vi "Stop Tracking.vi"(8 "error in (no error)":errorcluster, 10 "Tracker Type":refnum<class "Data Tracker Msg.lvclass">, 11 "Data Tracker in":refnum<class "Data Tracker.lvclass">) -> (0 "error out":errorcluster, 1 "Start Time":timestamp, 2 "Data":refnum<class "Data.lvclass">[](array[class]), 3 "Data Tracker out":refnum<class "Data Tracker.lvclass">, 5 "Duration(s)":dbl)   [LabVIEW 2020, in "Data Tracker.lvlib" / "Data Tracker.lvclass"]
doc: "Clean up the data assosicated with 'Tracker Type', stop tracking the data and cancel subscriptions on the Publisher actor if needed.\nReturn the tracked Data, the Start Time and the tracking Duration."
uses:
  Data Tracker.lvclass
  Messages for this Actor/Data Tracker Msg/Data Tracker Msg.lvclass
  PPL/HDH.Data.Generic.lvlibp/Data.lvclass
  PPL/HDH.Actor Framework.Core.Actor.lvlibp/1abvi3w/vi.lib/ActorFramework/Message Enqueuer/Message Priority.ctl
  Data Tracker.lvclass/Data Tracker.ctl
  PPL/HDH.Actor Framework.Core.Publisher.lvlibp/Publisher Messages/Unsubscribe Msg/Unsubscribe Msg.lvclass
  PPL/HDH.Actor Framework.Core.Actor.lvlibp/1abvi3w/vi.lib/ActorFramework/Message Enqueuer/Message Enqueuer.lvclass
  C:/Current projects/WS/PPL/HDH.Actor Framework.Core.Actor.lvlibp/1abvi3w/vi.lib/ActorFramework/Actor/Actor.lvclass
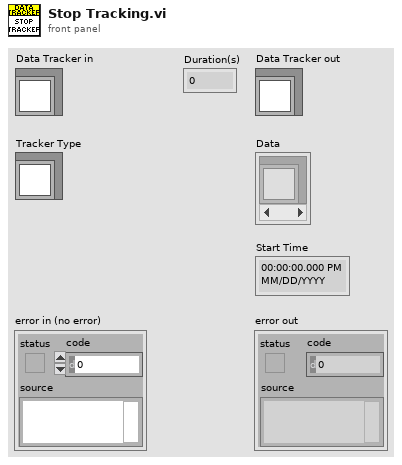
[diagram p1: front panel]
types:
  T1 = typedef "HDH.Actor Framework.Core.Actor.lvlibp/Message Enqueuer.lvclass/Message Priority.ctl" = enum16{"Low", "Normal", "High"}
  T2 = typedef "Data Tracker.lvlib/Data Tracker.lvclass/Ctl_Tracker Element.ctl" = cluster{"Tracker Type":refnum<class "Data Tracker Msg.lvclass">, "Subscriptions":refnum<class "Data.lvclass">[], "Data":refnum<class "Data.lvclass">[], "Size":u32, "Start Time":timestamp}
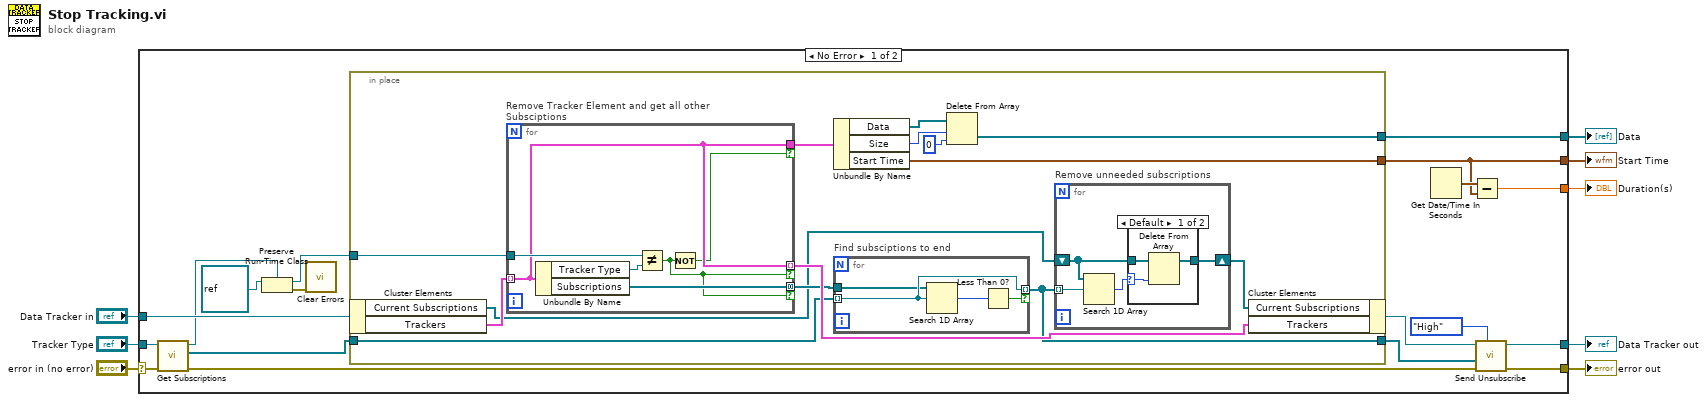
[diagram p0: block diagram]
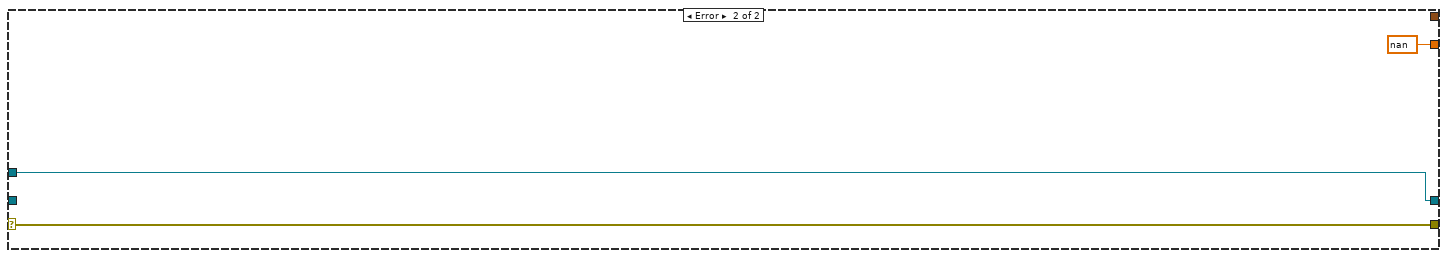
[diagram p3: hidden frame]
diagram:
  n1 = case shown="No Error" "error in (no error)" {
    selector: "error in (no error)" -> [w26 w61]
    tunnel: [w15 w61] -> w7
    tunnel: [w18 w60] -> w5
    tunnel: "Data Tracker in" -> [w24 w60]
    tunnel: "Tracker Type" -> [w22 _]
    tunnel: [w12 _] -> w3
    tunnel: [w10 _] -> w2
    tunnel: [w9 nan] -> w1
    frame No Error {
      n2 = call-dynamic "Get Subscriptions.vi"("error in (no error)"=w26, "Data Tracker Msg in"=w22) -> ("error out"=w16:errorcluster, "Subscriptions"=w20:refnum<class "Data.lvclass">[], "Data Tracker Msg out"=w21:refnum<class "Data Tracker Msg.lvclass">)  [unwired: 7 in]
      n3 = Preserve Run-Time Class(object in=refnum<class> refnum ("LabVIEW Object"), 2:w21) -> (object out=w23:refnum<class "Data Tracker Msg.lvclass">, error out=w25:errorcluster)  [unwired: 1 in]
      n4 = call <vilib>:"Clear Errors.vi"("error in (no error)"=w25) -> ()  [unwired: 5 in, 2 out]
      n5 = in-place {
        in-place-border: w23 -> [w39]
        in-place-border: w20 -> [w37]
        in-place-border: [w33] -> w14
        in-place-border: [w28] -> w12
        in-place-border: [w27] -> w10
        n6 = in-place-cluster #1(w24) -> ("Current Subscriptions"=w35:refnum<class "Data.lvclass">[], "Trackers"=w40:T2[])
        n7 = for "Remove Tracker Element and get all other Subsciptions" {
          tunnel: w40 -> [w55] mode=indexing
          tunnel: w39 -> [w58]
          tunnel: [w55] -> w38 mode=indexing if=w53
          tunnel: [w56] -> w36 mode=concatenating if=w53
          tunnel: [w55] -> w32 if=w54
          n8 = Unbundle By Name(w55) -> ("Tracker Type"=w57:refnum<class "Data Tracker Msg.lvclass">, "Subscriptions"=w56:refnum<class "Data.lvclass">[])
          n9 = Not Equal?(x=w58, y=w57) -> (x != y?=w53:bool)
          n10 = Not(x=w53) -> (.not. x?=w54:bool)
        }
        n11 = Unbundle By Name(w32) -> ("Data"=w31:refnum<class "Data.lvclass">[], "Size"=w29:u32, "Start Time"=w27:timestamp)
        n12 = for "Find subsciptions to end" {
          tunnel: w37 -> [w52] mode=indexing
          tunnel: [w52] -> w33 mode=indexing if=w51
          tunnel: w36 -> [w49]
          n13 = Search 1D Array(1D array=w49, element=w52) -> (index of element=w50:i32)  [unwired: 1 in]
          n14 = Less Than 0?(x=w50) -> (x < 0?=w51:bool)
        }
        n15 = Delete From Array(array=w31, length=w29, index=0) -> (deleted portion=w28:refnum<class "Data.lvclass">[])  [unwired: 1 out]
        n16 = for "Remove unneeded subscriptions" {
          shift-right: [w42] -> w34
          shift-left: w35 -> [w41]
          tunnel: w33 -> [w44] mode=indexing
          n17 = Search 1D Array(1D array=w41, element=w44) -> (index of element=w43:i32)  [unwired: 1 in]
          n18 = case shown="Default" w43 {
            selector: w43 -> [w46 _]
            tunnel: [w45 w48] -> w42
            tunnel: w41 -> [w47 w48]
            frame Default {
              n19 = Delete From Array(array=w47, index=w46) -> (array with subset deleted=w45:refnum<class "Data.lvclass">[])  [unwired: 1 in, 1 out]
            }
            frame -1 {
            }
          }
        }
        n20 = in-place-cluster #1("Current Subscriptions"=w34, "Trackers"=w38) -> (w19:refnum<class "Data Tracker.lvclass">)
      }
      n21 = Get Date/Time In Seconds() -> (seconds since 1Jan1904=w11:timestamp)
      n22 = Subtract(x=w11, y=w10) -> (x-y=w9:dbl)
      n23 = call "Send Unsubscribe.vi"("Message Priority (High)"=Message_Priority."High", "error in (no error)"=w16, "Data Array"=w14, "Actor in"=w19) -> ("error out"=w15:errorcluster, "Actor out"=w18:refnum<class "Data Tracker.lvclass">)  [unwired: 6 in]
    }
    frame Error {
    }
  }
  "error out" <- w7
  "Data Tracker out" <- w5
  "Data" <- w3
  "Start Time" <- w2
  "Duration(s)" <- w1
